vi "StringS_request.vi"(8 "error in (no error)":errorcluster, 10 "SQL request":string, 11 "DB_SQLite in":refnum<class "DB_SQLite.lvclass">) -> (0 "error out":errorcluster, 1 "Column Names":string[](array[string]), 2 "Result Set":string[][](table) caption="Result Set (from first statement with results)", 3 "DB_SQLite out":refnum<class "DB_SQLite.lvclass">)   [LabVIEW 2018, in "DB_SQLite.lvclass"]
uses:
  DB_SQLite.lvclass
  <vilib>/drjdpowell/SQLite Library/SQL Connection/Execute SQL.vi
  <vilib>/drjdpowell/SQLite Library/SQLite.lvlib
  <vilib>/drjdpowell/SQLite Library/SQL Connection/Connection.lvclass
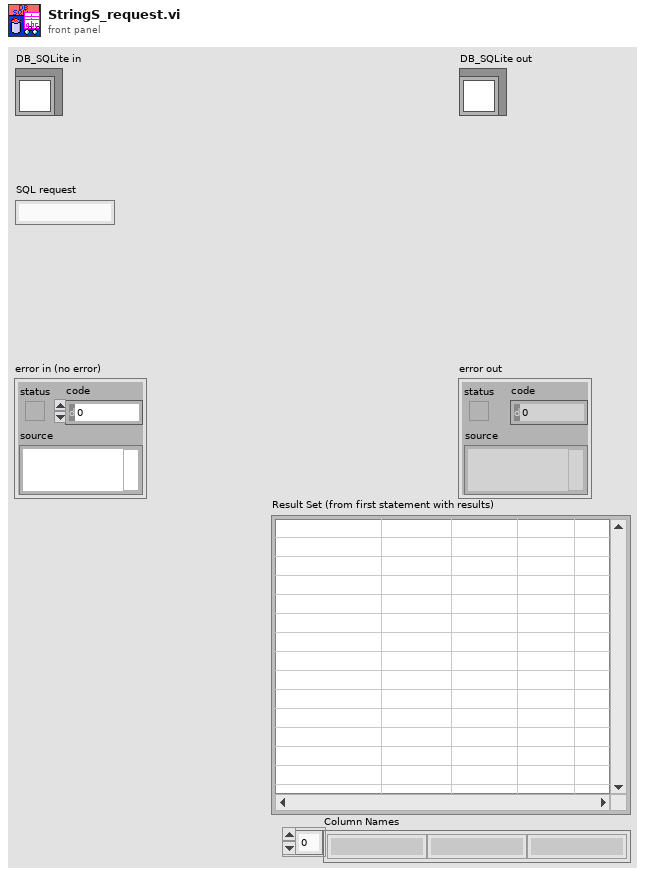
[diagram p1: front panel]
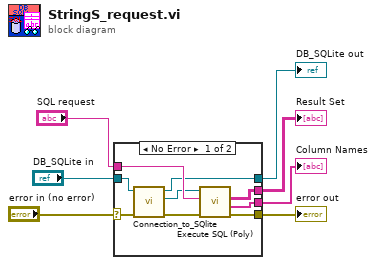
[diagram p0: block diagram]
diagram:
  n1 = case shown="No Error" "error in (no error)" {
    selector: "error in (no error)" -> [w9 w17]
    tunnel: "DB_SQLite in" -> [w12 w18]
    tunnel: [w11 w18] -> w5
    tunnel: [w16 _] -> w4
    tunnel: "SQL request" -> [w15 _]
    tunnel: [w13 w17] -> w2
    tunnel: [w14 _] -> w1
    frame No Error {
      n2 = call "Connection_to_SQlite.vi"("error in (no error)"=w9, "DB_SQLite in"=w12) -> ("error out"=w8:errorcluster, "SQlite connection"=w10:refnum<class "Connection.lvclass">, "DB_SQLite out"=w11:refnum<class "DB_SQLite.lvclass">)  [unwired: 7 in]
      n3 = call-poly <vilib>:"Execute SQL (Poly).vi"("error in (no error)"=w8, "SQL"=w15, "SQLite Connection in"=w10) -> ("error out"=w13:errorcluster, "Column Names"=w14:string[], "Result Set"=w16:string[][])  [unwired: 5 in, 1 out]
    }
    frame Error {
    }
  }
  "error out" <- w2
  "DB_SQLite out" <- w5
  "Result Set" <- w4
  "Column Names" <- w1
